vi "SampleSubVI.vi"(0 "task out":refnum<k21> caption="任务输出", 1 "Courter 1":refnum<k21> caption="任务/通道输入1", 3 "Courter 4":refnum<k21> caption="任务/通道输入4", 4 "Courter 2":refnum<k21> caption="任务/通道输入2", 6 "数组":sgl[](array[numeric]), 10 "Courter 3":refnum<k21> caption="任务/通道输入3", 15 "Courter 5":refnum<k21> caption="任务/通道输入5") -> (7 "压力信号":dbl[](array[numeric]), 9 "一级轴向力":dbl[](array[numeric]), 12 "vmic反馈数据":sgl[](array[numeric]), 13 "力臂":dbl[](array[numeric]), 14 "AngleSample":dbl[](array[numeric]), 16 "加速度信号":dbl[](array[numeric]), 19 "一二级侧向力矩":dbl[](array[numeric]), 21 "F_outrange":bool[](array[boolean]), 24 "error out":errorcluster, 25 "一二级侧向位移":dbl[](array[numeric]), 27 "一级侧向力反馈":dbl[](array[numeric]))   [LabVIEW 2020]
uses:
  <vilib>/DAQmx/read.llb/DAQmx Read (Counter DBL 1Chan 1Samp).vi
  <vilib>/DAQmx/read.llb/DAQmx Read (Analog 1D DBL NChan 1Samp).vi
  <vilib>/DAQmx/miscellaneous.llb/DAQmx Fill In Error Info.vi
  <vilib>/Analysis/NI_AALBase.lvlib
  <vilib>/Analysis/3filter.llb/Filter Passband Type.ctl
  <vilib>/Analysis/3filter.llb/Butterworth Filter (DBL).vi
panel:
  out "元素 2":dbl
  out "元素":dbl
  out "二级轴向力":dbl[](array[numeric])
  out "二级侧向力反馈 2":dbl[](array[numeric])
  out "data":dbl[](array[numeric]) caption="数据" format="%0.2f"
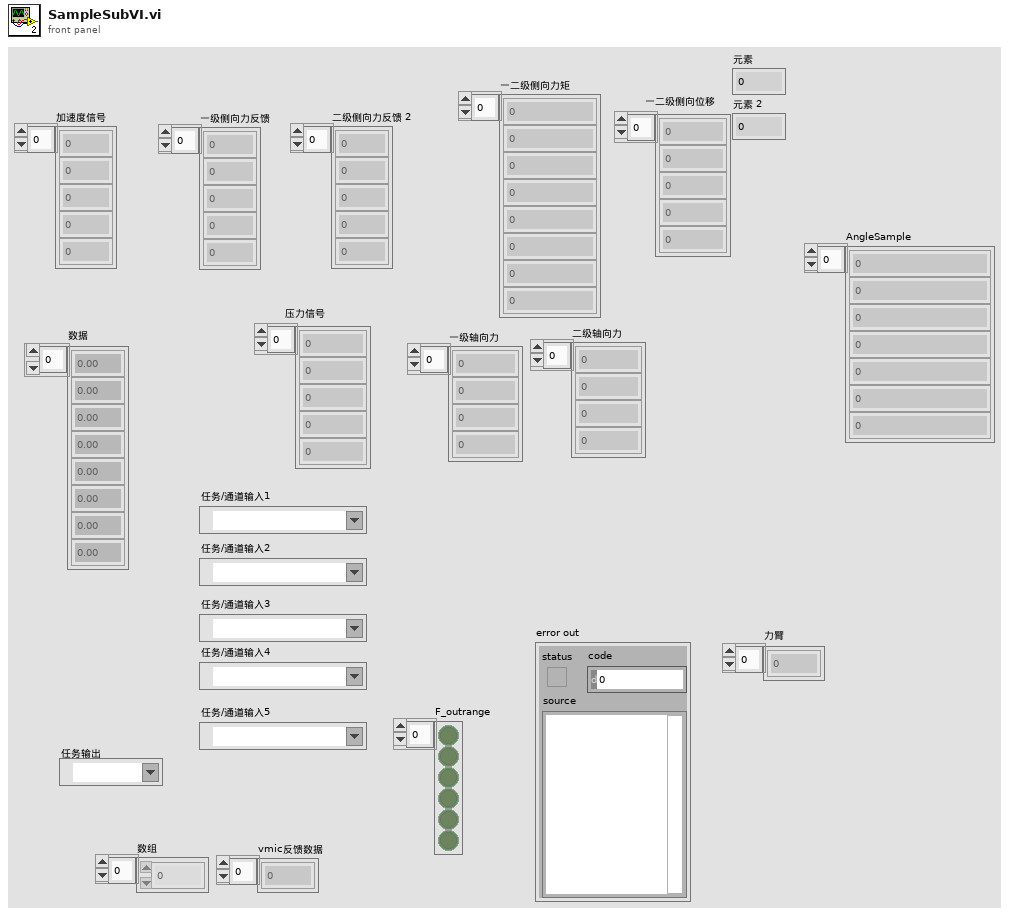
[diagram p1: front panel]
types:
  T1 = typedef "NI_AALBase.lvlib/Filter Passband Type.ctl" = enum32{"Lowpass", "Highpass", "Bandpass", "Bandstop"}
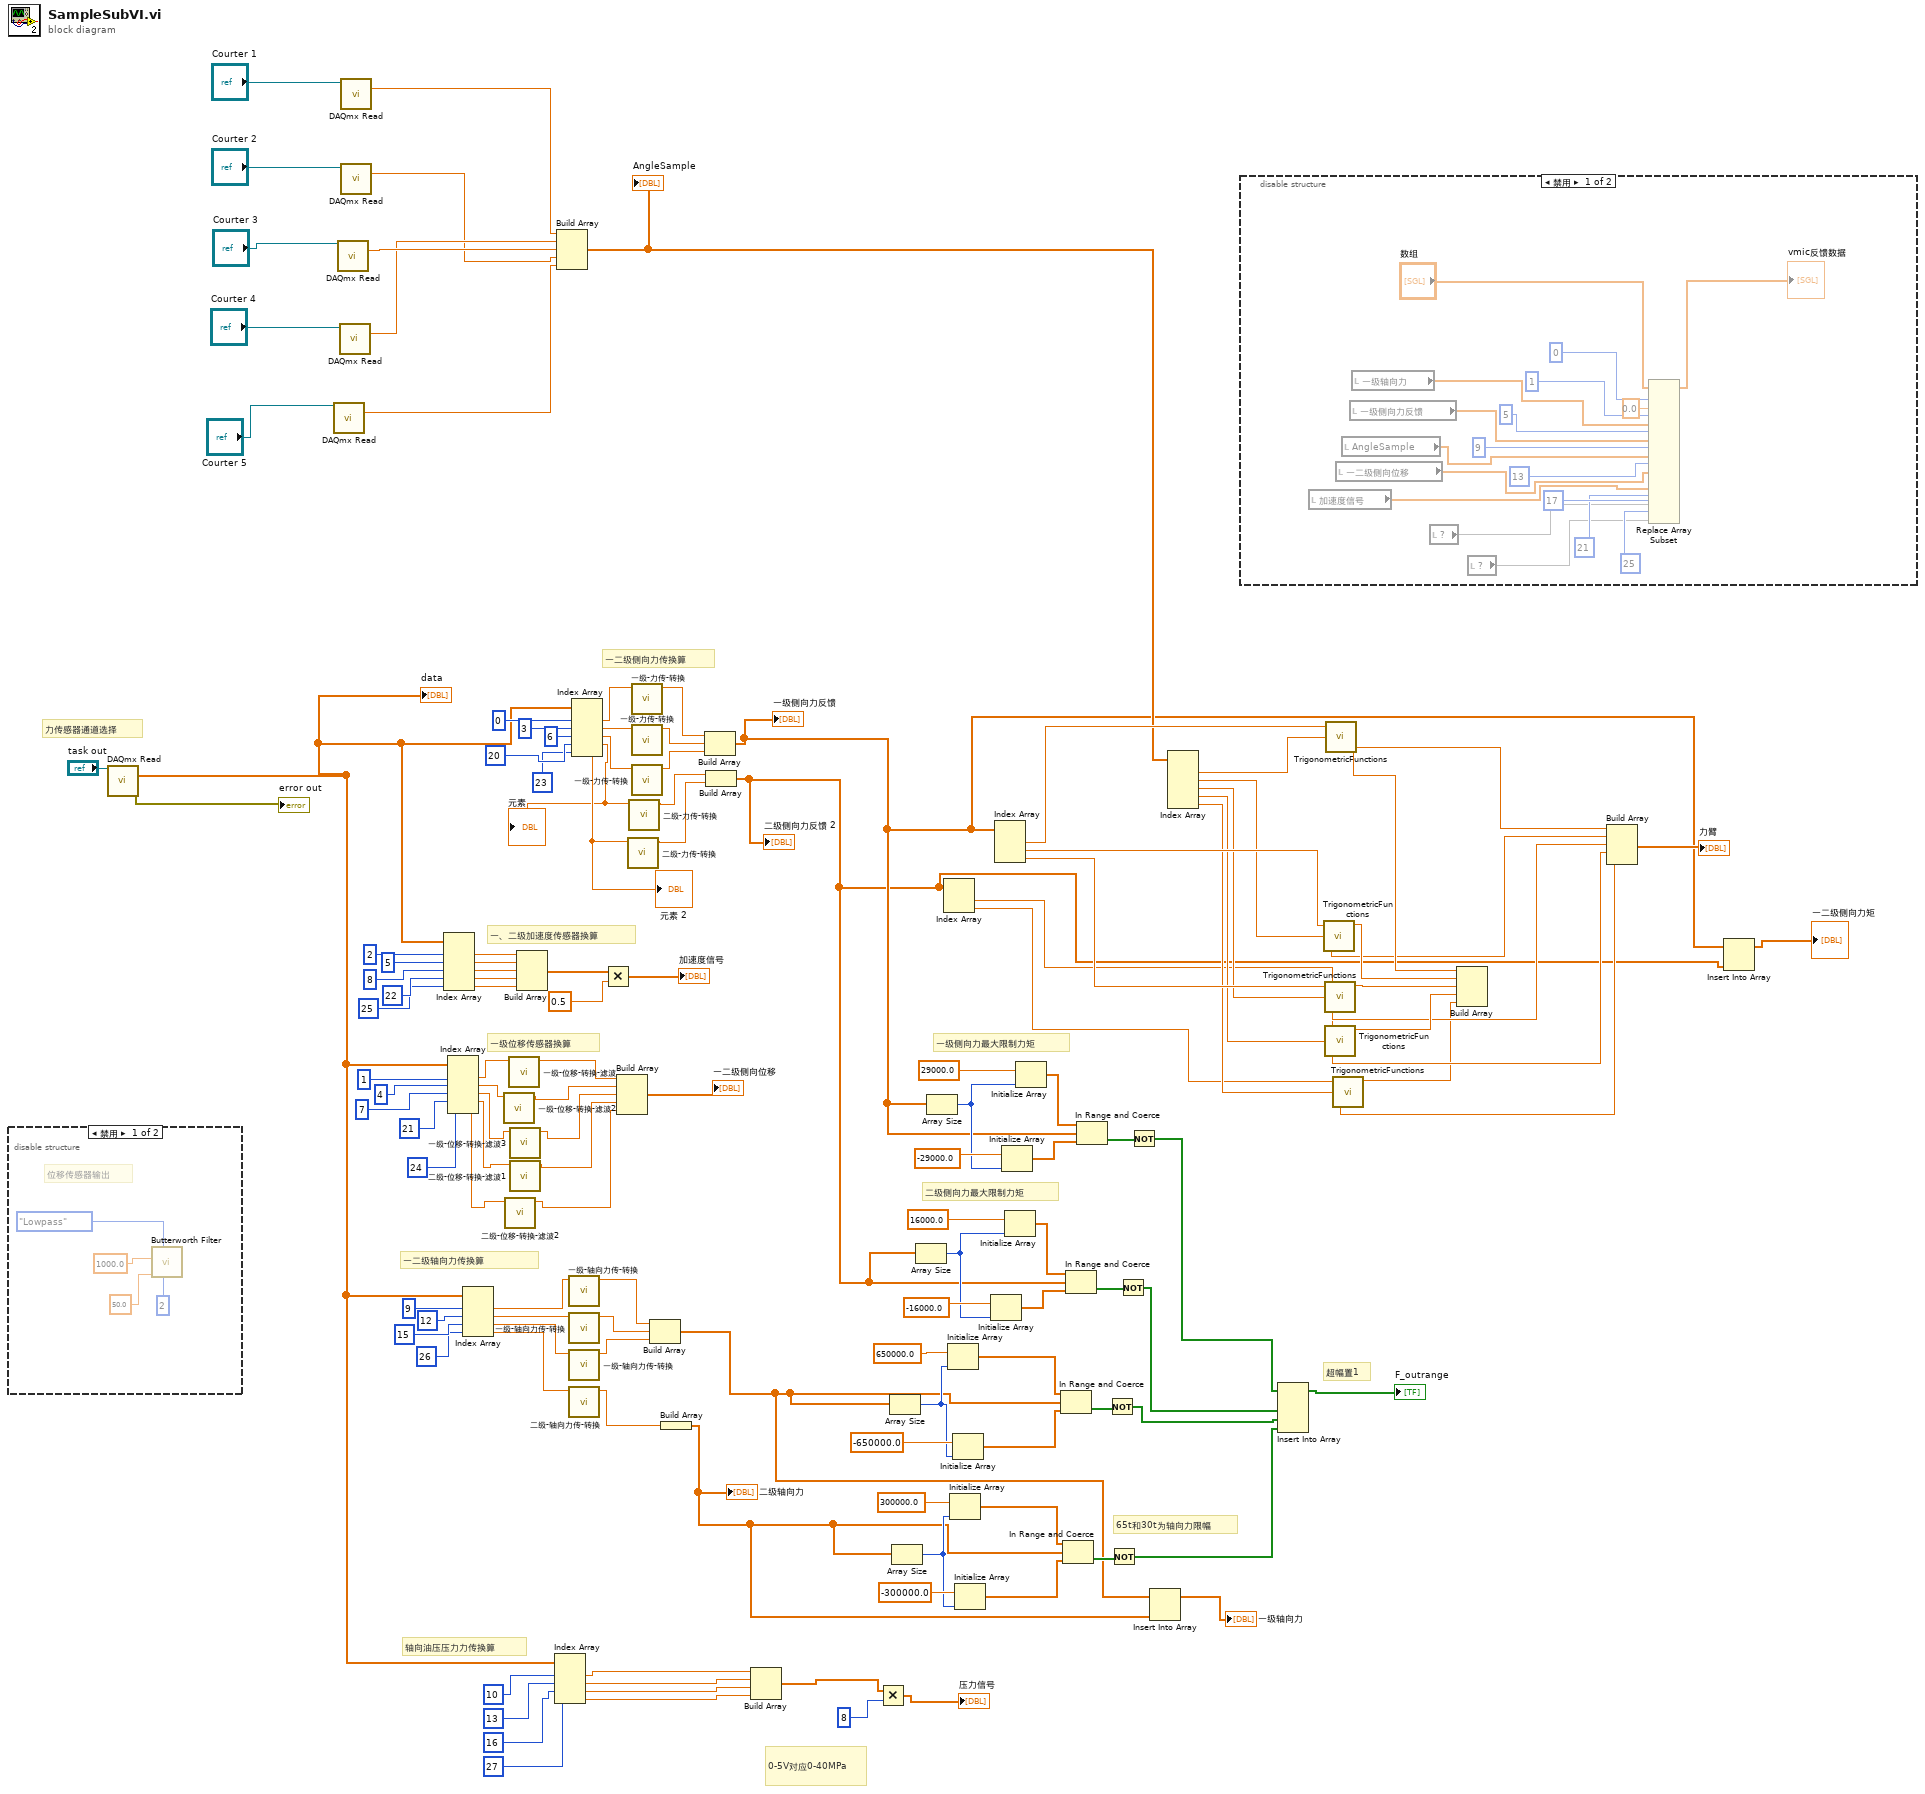
[diagram p0: block diagram]
diagram:
  # "二级侧向力最大限制力矩"
  # "轴向油压压力力传换算"
  # "0-5V对应0-40MPa"
  # "65t和30t为轴向力限幅"
  # "一级位移传感器换算"
  # "一二级侧向力传换算"
  # "一、二级加速度传感器换算"
  # "力传感器通道选择"
  # "一二级轴向力传换算"
  # "超幅置1"
  # "一级侧向力最大限制力矩"
  n1 = disable-structure shown="禁用" {
    frame Disabled {
      # "位移传感器输出"
      n2 = call-poly <vilib>:"Butterworth Filter.vi"("order"=2, "filter type"=Filter_Passband_Type."Lowpass", "low cutoff freq: fl"=50.0, "sampling freq: fs"=1000.0) -> ()  [unwired: 4 in, 2 out]
    }
    frame Enabled {
    }
  }
  n3 = call-poly <vilib>:"DAQmx Read.vi"("task/channels in"="task out") -> ("data"=w65:dbl[], "error out"=→"error out":errorcluster)  [unwired: 12 in, 1 out]
  "data" <- w65
  n4 = call-poly <vilib>:"DAQmx Read.vi"("task/channels in"="Courter 5") -> ("data"=w79:dbl)  [unwired: 12 in, 2 out]
  n5 = call-poly <vilib>:"DAQmx Read.vi"("task/channels in"="Courter 3") -> ("data"=w86:dbl)  [unwired: 12 in, 2 out]
  n6 = call-poly <vilib>:"DAQmx Read.vi"("task/channels in"="Courter 4") -> ("data"=w85:dbl)  [unwired: 12 in, 2 out]
  n7 = call-poly <vilib>:"DAQmx Read.vi"("task/channels in"="Courter 1") -> ("data"=w94:dbl)  [unwired: 12 in, 2 out]
  n8 = call-poly <vilib>:"DAQmx Read.vi"("task/channels in"="Courter 2") -> ("data"=w84:dbl)  [unwired: 12 in, 2 out]
  n9 = Index Array(array=w65, index #1=2 ("索引"), index #2=5 ("索引"), index #3=8 ("索引"), index #4=22 ("索引"), index #5=25 ("索引")) -> (element #1=w127:dbl, element #2=w126:dbl, element #3=w125:dbl, element #4=w124:dbl, element #5=w70:dbl)
  n10 = Index Array(array=w65, index #1=1 ("索引"), index #2=4 ("索引"), index #3=7 ("索引"), index #4=21 ("索引"), index #5=24 ("索引")) -> (element #1=w133:dbl, element #2=w68:dbl, element #3=w66:dbl, element #4=w8:dbl, element #5=w9:dbl)
  n11 = Index Array(array=w65, index #1=9 ("索引"), index #2=12 ("索引"), index #3=15 ("索引"), index #4=26 ("索引")) -> (element #1=w39:dbl, element #2=w38:dbl, element #3=w37:dbl, element #4=w36:dbl)
  n12 = call "一级-位移-转换-滤波2.vi"("Waveform"=w68) -> ("Filtered x"=w69:dbl)  [unwired: 10 in]
  n13 = call "二级-位移-转换-滤波2.vi"("Waveform"=w9) -> ("Filtered x"=w10:dbl)  [unwired: 10 in]
  n14 = call "一级-位移-转换-滤波.vi"("Waveform"=w133) -> ("Filtered x"=w82:dbl)  [unwired: 10 in]
  n15 = call "一级-位移-转换-滤波3.vi"("Waveform"=w66) -> ("Filtered x"=w67:dbl)  [unwired: 10 in]
  n16 = call "二级-位移-转换-滤波1.vi"("Waveform"=w8) -> ("Filtered x"=w7:dbl)  [unwired: 10 in]
  n17 = Build Array(w127, w126, w125, w124, w70) -> (w128:dbl[])
  n18 = Index Array(array=w65, index #1=10 ("索引"), index #2=13 ("索引"), index #3=16 ("索引"), index #4=27 ("索引")) -> (element #1=w50:dbl, element #2=w49:dbl, element #3=w48:dbl, element #4=w47:dbl)
  n19 = Build Array(w94, w85, w86, w84, w79) -> (w93:dbl[])
  "AngleSample" <- w93
  n20 = call "一级-轴向力传-转换.vi"("Waveform"=w39) -> ("Filtered x"=w35:dbl)  [unwired: 10 in]
  n21 = call "一级-轴向力传-转换.vi"("Waveform"=w38) -> ("Filtered x"=w34:dbl)  [unwired: 10 in]
  n22 = call "一级-轴向力传-转换.vi"("Waveform"=w37) -> ("Filtered x"=w33:dbl)  [unwired: 10 in]
  n23 = call "二级-轴向力传-转换.vi"("Waveform"=w36) -> ("Filtered x"=w14:dbl)  [unwired: 10 in]
  n24 = Index Array(array=w65, index #1=0 ("索引"), index #2=3 ("索引"), index #3=6 ("索引"), index #4=20 ("索引"), index #5=23 ("索引")) -> (element #1=w81:dbl, element #2=w75:dbl, element #3=w73:dbl, element #4=w40:dbl, element #5=w41:dbl)
  "元素" <- w40
  "元素 2" <- w41
  n25 = Multiply(x=w128, y=0.5) -> (x*y=→"加速度信号":dbl[])
  n26 = Build Array(w82, w69, w67, w7, w10) -> (→"一二级侧向位移":dbl[])
  n27 = call "二级-力传-转换.vi"("Waveform"=w41) -> ("Filtered x"=w31:dbl)  [unwired: 10 in]
  n28 = call "二级-力传-转换.vi"("Waveform"=w40) -> ("Filtered x"=w32:dbl)  [unwired: 10 in]
  n29 = call "一级-力传-转换.vi"("Waveform"=w81) -> ("Filtered x"=w80:dbl)  [unwired: 10 in]
  n30 = call "一级-力传-转换.vi"("Waveform"=w75) -> ("Filtered x"=w74:dbl)  [unwired: 10 in]
  n31 = call "一级-力传-转换.vi"("Waveform"=w73) -> ("Filtered x"=w72:dbl)  [unwired: 10 in]
  n32 = Build Array(w35, w34, w33) -> (w2:dbl[])
  n33 = Build Array(w14) -> (w1:dbl[])
  "二级轴向力" <- w1
  n34 = Build Array(w80, w74, w72) -> (w5:dbl[])
  "一级侧向力反馈" <- w5
  n35 = Build Array(w32, w31) -> (w4:dbl[])
  "二级侧向力反馈 2" <- w4
  n36 = Build Array(w50, w49, w48, w47) -> (w12:dbl[])
  n37 = Multiply(x=w12, y=8) -> (x*y=→"压力信号":dbl[])
  n38 = Array Size(array=w2) -> (size(s)=w57:i32)
  n39 = Array Size(array=w1) -> (size(s)=w15:i32)
  n40 = Array Size(array=w4) -> (size(s)=w23:i32)
  n41 = Array Size(array=w5) -> (size(s)=w56:i32)
  n42 = Index Array(array=w4) -> (element #1=w29:dbl, element #2=w30:dbl)  [unwired: 2 in]
  n43 = Initialize Array(650000.0, w57) -> (w58:dbl[])
  n44 = Initialize Array(300000.0, w15) -> (w16:dbl[])
  n45 = Initialize Array(-650000.0, w57) -> (w59:dbl[])
  n46 = Initialize Array(-300000.0, w15) -> (w17:dbl[])
  n47 = Initialize Array(-16000.0, w23) -> (w24:dbl[])
  n48 = Index Array(array=w5) -> (element #1=w113:dbl, element #2=w112:dbl, element #3=w111:dbl)  [unwired: 3 in]
  n49 = Initialize Array(-29000.0, w56) -> (w99:dbl[])
  n50 = Initialize Array(16000.0, w23) -> (w26:dbl[])
  n51 = Initialize Array(29000.0, w56) -> (w101:dbl[])
  n52 = In Range and Coerce(upper limit=w58, x=w2, lower limit=w59) -> (In Range?=w116:bool[])  [unwired: 1 out]
  n53 = In Range and Coerce(upper limit=w16, x=w1, lower limit=w17) -> (In Range?=w20:bool[])  [unwired: 1 out]
  n54 = In Range and Coerce(upper limit=w26, x=w4, lower limit=w24) -> (In Range?=w28:bool[])  [unwired: 1 out]
  n55 = In Range and Coerce(upper limit=w101, x=w5, lower limit=w99) -> (In Range?=w137:bool[])  [unwired: 1 out]
  n56 = Not(x=w116) -> (.not. x?=w22:bool[])
  n57 = Not(x=w20) -> (.not. x?=w13:bool[])
  n58 = Not(x=w28) -> (.not. x?=w21:bool[])
  n59 = Not(x=w137) -> (.not. x?=w115:bool[])
  n60 = Insert Into Array(array=w2, new element=w1) -> (→"一级轴向力":dbl[])  [unwired: 1 in]
  n61 = Index Array(array=w93) -> (element #1=w110:dbl, element #2=w109:dbl, element #3=w108:dbl, element #4=w107:dbl, element #5=w53:dbl)  [unwired: 5 in]
  n62 = disable-structure shown="禁用" {
    frame Disabled {
      n63 = local read "加速度信号"() -> (w147:dbl[])
      n64 = local read "一二级侧向位移"() -> (w148:dbl[])
      n65 = local read "AngleSample"() -> (w149:dbl[])
      n66 = local read "一级侧向力反馈"() -> (w150:dbl[])
      n67 = local read "一级轴向力"() -> (w151:dbl[])
      n68 = local read item#-1() -> (w146)
      n69 = local read item#-1() -> (w145)
      n70 = Replace Array Subset(array="数组", new element #1=sgl 0.0 ("新元素/子数组"), index #1=0 ("索引"), new element #2=w151, index #2=1 ("索引"), new element #3=w150, index #3=5 ("索引"), new element #4=w149, index #4=9 ("索引"), new element #5=w148, index #5=13 ("索引"), new element #6=w147, index #6=17 ("索引"), new element #7=w146, index #7=21 ("索引"), new element #8=w145, index #8=25 ("索引")) -> (→"vmic反馈数据":sgl[])
    }
    frame Enabled {
    }
  }
  n71 = Insert Into Array(array=w115, new element #1=w21, new element #2=w22, new element #3=w13) -> (→"F_outrange":bool[])  [unwired: 1 in]
  n72 = call "TrigonometricFunctions.vi"("摆角采样"=w109, "力采样N"=w112) -> ("力矩采样Nm"=w105:dbl, "力臂"=w91:dbl)  [unwired: 5 in]
  n73 = call "TrigonometricFunctions.vi"("摆角采样"=w108, "力采样N"=w111) -> ("力矩采样Nm"=w104:dbl, "力臂"=w90:dbl)  [unwired: 5 in]
  n74 = call "TrigonometricFunctions.vi"("摆角采样"=w107, "力采样N"=w29) -> ("力矩采样Nm"=w103:dbl, "力臂"=w89:dbl)  [unwired: 5 in]
  n75 = call "TrigonometricFunctions.vi"("摆角采样"=w110, "力采样N"=w113) -> ("力矩采样Nm"=w106:dbl, "力臂"=w92:dbl)  [unwired: 5 in]
  n76 = call "TrigonometricFunctions.vi"("摆角采样"=w53, "力采样N"=w30) -> ("力矩采样Nm"=w52:dbl, "力臂"=w51:dbl)  [unwired: 5 in]
  n77 = Build Array(w106, w105, w104, w103, w52) -> ()  [unwired: 1 out]
  n78 = Build Array(w92, w91, w90, w89, w51) -> (→"力臂":dbl[])
  n79 = Insert Into Array(array=w5, new element=w4) -> (→"一二级侧向力矩":dbl[])  [unwired: 1 in]
